vi "GetAlarms.vi"(0 "Proccess in":refnum<class "Proccess.lvclass">, 11 "error in (no error)":errorcluster) -> (4 "Proccess out":refnum<class "Proccess.lvclass">, 6 "Alarm":bool, 8 "Warning":bool, 15 "error out":errorcluster)   [LabVIEW 2019, in "Proccess.lvclass"]
uses:
  Proccess.lvclass
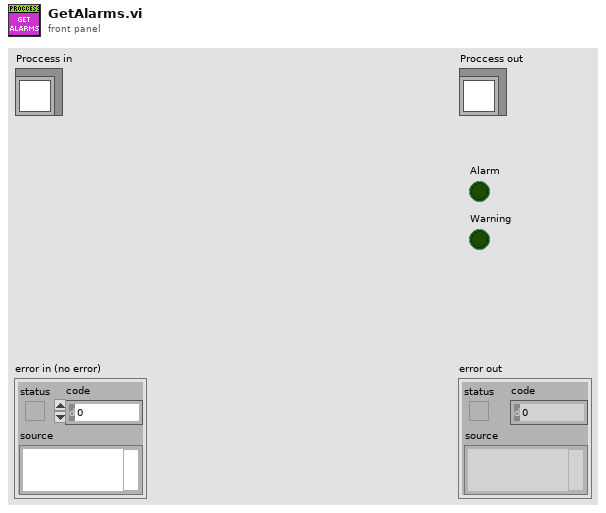
[diagram p1: front panel]
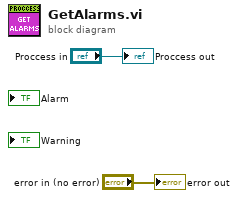
[diagram p0: block diagram]
diagram:
  "error out" <- "error in (no error)"
  "Proccess out" <- "Proccess in"
